vi "Send Command.vi"(8 "error in (no error)":errorcluster, 9 "command delay (ms)":u32=100, 10 "Command":string, 11 "LibreVNA in":refnum<class "LibreVNA.lvclass">) -> (0 "error out":errorcluster, 1 "bytes written":i32, 3 "LibreVNA out":refnum<class "LibreVNA.lvclass">)   [LabVIEW 2023, in "LibreVNA.lvclass"]
uses:
  LibreVNA.lvclass
  <userlib>/_OpenG.lib/time/time.llb/openg_time.lvlib
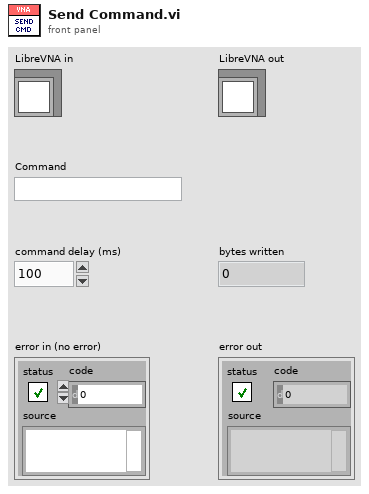
[diagram p1: front panel]
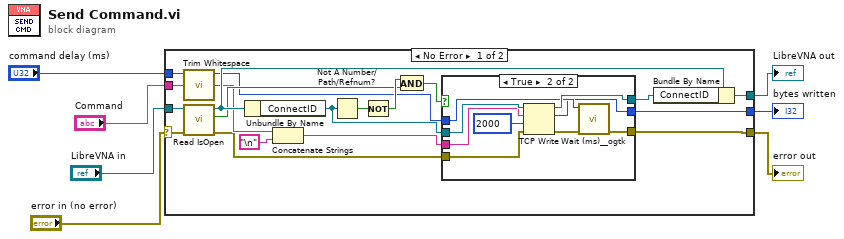
[diagram p0: block diagram]
diagram:
  n1 = case shown="No Error" "error in (no error)" {
    selector: "error in (no error)" -> [w20 w38]
    tunnel: [w11 w38] -> w6
    tunnel: [w13 w37] -> w4
    tunnel: "LibreVNA in" -> [w25 w37]
    tunnel: "Command" -> [w18 _]
    tunnel: "command delay (ms)" -> [w9 _]
    tunnel: [w8 _] -> w1
    frame No Error {
      n2 = call <vilib>:"Trim Whitespace.vi"("string"=w18) -> ("trimmed string"=w17:string)  [unwired: 1 in]
      n3 = call-dynamic "Read IsOpen.vi"("error in (no error)"=w20, "LibreVNA in"=w25) -> ("error out"=w14:errorcluster, "IsOpen"=w21:bool, "LibreVNA out"=w24:refnum<class "LibreVNA.lvclass">)  [unwired: 7 in]
      n4 = Unbundle By Name(w24) -> ("ConnectID"=w19:refnum<k5>)
      n5 = Concatenate Strings(w17, "\n") -> (w16:string)
      n6 = Not A Number/Path/Refnum?(number/path/refnum=w19) -> (NaN/Path/Refnum?=w23:bool)
      n7 = Not(x=w23) -> (.not. x?=w22:bool)
      n8 = And(x=w22, y=w21) -> (x .and. y?=w10:bool)
      n9 = case shown="True" w10 {
        tunnel: w19 -> [w27 w36]
        tunnel: w16 -> [_ w35]
        tunnel: w14 -> [w26 w34]
        tunnel: [w27 w32] -> w12
        tunnel: [w26 w30] -> w11
        tunnel: w9 -> [_ w29]
        tunnel: [_ w28] -> w8
        frame False {
        }
        frame True {
          n10 = TCP Write(connection ID=w36, data in=w35, error in (no error)=w34, 9:2000 ("timeout ms (25000)")) -> (connection ID out=w32:refnum<k5>, bytes written=w28:i32, error out=w31:errorcluster)
          n11 = call <userlib>:"Wait (ms)__ogtk.vi"("error in (no error)"=w31, "milliseconds to wait"=w29) -> ("error out"=w30:errorcluster)  [unwired: 8 in, 1 out]
        }
      }
      n12 = Bundle By Name(cluster=w24, "ConnectID"=w12) -> (w13:refnum<class "LibreVNA.lvclass">)
    }
    frame Error {
    }
  }
  "error out" <- w6
  "LibreVNA out" <- w4
  "bytes written" <- w1
